vi "Generate Calibrated Sine Waveform.vi"(0 "TSM context":T1, 5 "Frequency (Hz)":dbl, 7 "dB SPL":dbl, 9 "Sampling Rate (Hz)":dbl, 11 "error in (no error)":errorcluster, 12 "Samples per channel":dbl) -> (4 "Per-Site Waveforms Out":waveform(dbl)[](array[waveform]), 6 "Per Site Amplitude (V)":dbl[](array[numeric]), 15 "error out":errorcluster)   [LabVIEW 2020]
doc: "This VI helps to get the sine wave for each site in desired frequency"
uses:
  <vilib>/NI_TestStand_SemiconductorModule/NI_TestStand_Semiconductor_Module.lvlibp/PinMap/General/SemiconductorModuleContext.ctl
  <vilib>/measure/NI_MABase.lvlib
  <vilib>/NI_TestStand_SemiconductorModule/NI_TestStand_Semiconductor_Module.lvlibp
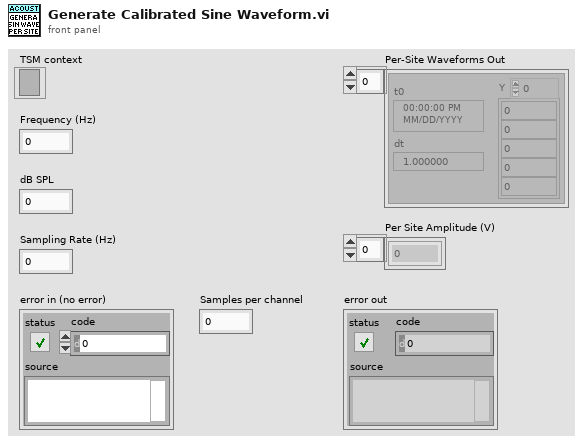
[diagram p1: front panel]
types:
  T1 = typedef "NI_TestStand_Semiconductor_Module.lvlibp/SemiconductorModuleContext.ctl" = refnum<k7>
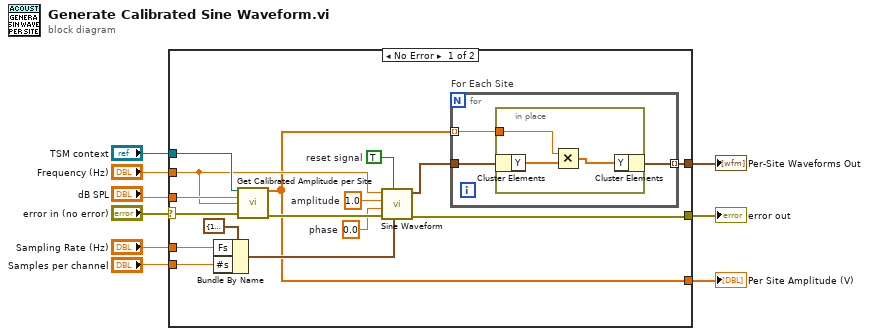
[diagram p0: block diagram]
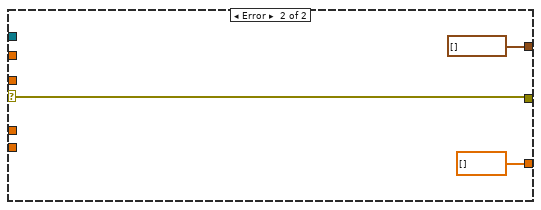
[diagram p2: hidden frame]
diagram:
  n1 = case shown="No Error" "error in (no error)" {
    selector: "error in (no error)" -> [w25 w34]
    tunnel: [w23 w34] -> w8
    tunnel: "dB SPL" -> [w22 _]
    tunnel: "TSM context" -> [w21 _]
    tunnel: "Frequency (Hz)" -> [w20 _]
    tunnel: "Sampling Rate (Hz)" -> [w18 _]
    tunnel: "Samples per channel" -> [w17 _]
    tunnel: [w11 dbl[] [] ("Per Site Amplitude (V)")] -> w2
    tunnel: [w10 waveform(dbl)[] []] -> w1
    frame No Error {
      w13 = 1.0  # amplitude
      w14 = 0.0  # phase
      w15 = TRUE  # reset signal
      n2 = Bundle By Name(cluster=cluster{"Fs":dbl, "#s":dbl} {"Fs"=1000.0, "#s"=1000.0} ("sampling info"), "Fs"=w18, "#s"=w17) -> (w16:cluster{"Fs":dbl, "#s":dbl})
      n3 = call "Get Calibrated Amplitude per Site.vi"("TSM context"=w21, "dB SPL"=w22, "Frequency (Hz)"=w20, "error in (no error)"=w25) -> ("Per Site Amplitude (V)"=w11:dbl[], "error out"=w24:errorcluster)  [unwired: 9 in, 1 out]
      n4 = call <vilib>:"Sine Waveform.vi"("sampling info"=w16, "reset signal"=w15, "error in (no error)"=w24, "phase"=w14, "amplitude"=w13, "frequency"=w20) -> ("error out"=w23:errorcluster, "signal out"=w12:waveform(dbl))  [unwired: 4 in]
      n5 = for "For Each Site" {
        tunnel: w12 -> [w28]
        tunnel: w11 -> [w27] mode=indexing
        tunnel: [w26] -> w10 mode=indexing
        n6 = in-place {
          in-place-border: w27 -> [w29]
          n7 = in-place-cluster #1(w28) -> ("Y"=w31:dbl[])
          n8 = Multiply(x=w29, y=w31) -> (x*y=w30:dbl[])
          n9 = in-place-cluster #1("Y"=w30) -> (w26:waveform(dbl))
        }
      }
    }
    frame Error {
    }
  }
  "error out" <- w8
  "Per Site Amplitude (V)" <- w2
  "Per-Site Waveforms Out" <- w1
